vi "Configure.vi"(8 "error in (no error)":errorcluster, 11 "Fetch Waveforms CFG in":refnum<class "Fetch Waveforms CFG.lvclass">) -> (0 "error out":errorcluster, 3 "Fetch Waveforms CFG out":refnum<class "Fetch Waveforms CFG.lvclass">)   [LabVIEW 2023, in "PXIe-4353.lvlib" / "Fetch Waveforms CFG.lvclass"]
uses:
  Fetch Waveforms CFG.lvclass
  Fetch Waveforms CFG.lvclass/Fetch Waveforms CFG.ctl
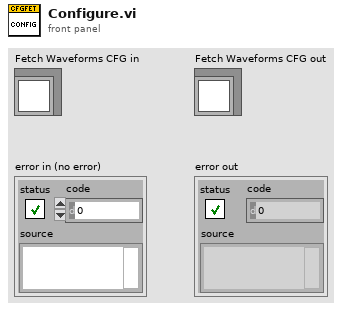
[diagram p1: front panel]
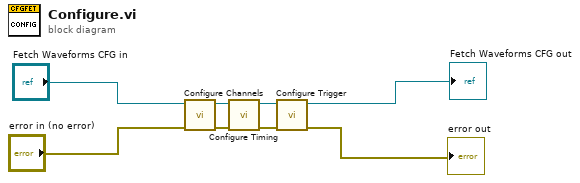
[diagram p0: block diagram]
diagram:
  n1 = call-dynamic "Configure Channels.vi"("error in (no error)"="error in (no error)", "Fetch Waveform CFG in"="Fetch Waveforms CFG in") -> ("error out"=w7:errorcluster, "Fetch Waveform CFG out"=w4:refnum<class "Fetch Waveforms CFG.lvclass">)  [unwired: 8 in]
  n2 = call-dynamic "Configure Timing.vi"("error in (no error)"=w7, "Thermometer DAQmx Config in"=w4) -> ("error out"=w5:errorcluster, "Thermometer DAQmx Config out"=w2:refnum<class "Fetch Waveforms CFG.lvclass">)  [unwired: 8 in]
  n3 = call-dynamic "Configure Trigger.vi"("error in (no error)"=w5, "Thermometer DAQmx Config in"=w2) -> ("error out"=→"error out":errorcluster, "Thermometer DAQmx Config out"=→"Fetch Waveforms CFG out":refnum<class "Fetch Waveforms CFG.lvclass">)  [unwired: 8 in]
